vi "StopGetPic.vi"() -> ()   [LabVIEW 2011]
panel:
  in  "Stop":bool
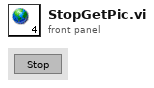
[diagram p1: front panel]
diagram:
